vi "Menu_Property Node.vi"(11 "Affected Items Out":T1) -> (3 "Menu Items To Add":T2(array[cluster]))   [LabVIEW 2023]
uses:
  top/BundleMagic.ctl
  controls/action enum.ctl
panel:
  out "element":refnum<vi>
  out "Enabled Status":enum8{"Enabled", "Disabled"}[](array[ring])
  out "Menu Item Display Name":string[](array[string])
  out "Position In Menu":T3(array[cluster])
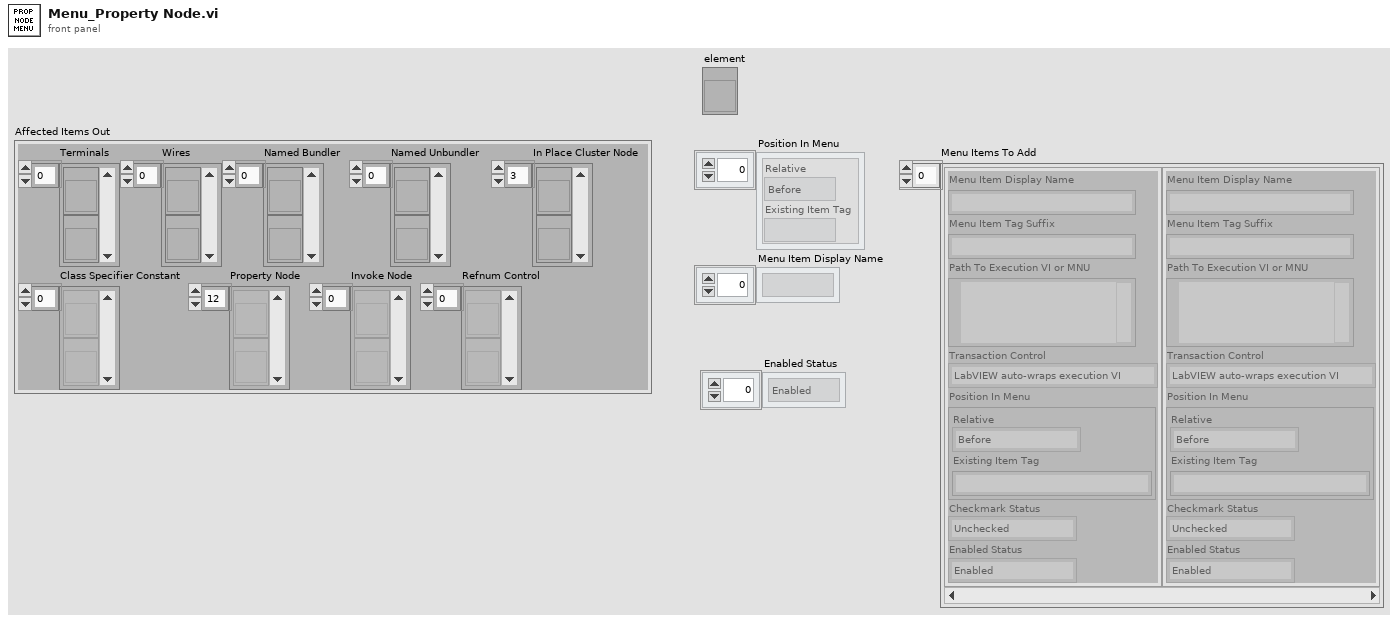
[diagram p1: front panel]
types:
  T1 = typedef "BundleMagic.ctl" = cluster{"Terminals":refnum<vi>[], "Wires":refnum<vi>[], "Named Bundler":refnum<vi>[], "Named Unbundler":refnum<vi>[], "In Place Cluster Node":refnum<vi>[], "Class Specifier Constant":refnum<vi>[], "Property Node":refnum<vi>[], "Invoke Node":refnum<vi>[], "Refnum Control":refnum<vi>[]}
  T2 = cluster{"Menu Item Display Name":string, "Menu Item Tag Suffix":string, "Path To Execution VI or MNU":path, "Transaction Control":enum8{"LabVIEW auto-wraps execution VI", "Execution VI will define if needed"}, "Position In Menu":cluster{"Relative":enum8{"Before", "Instead of", "After", "Into Submenu"}, "Existing Item Tag":string}, "Checkmark Status":enum8{"Unchecked", "Checked"}, "Enabled Status":enum8{"Enabled", "Disabled"}}[]
  T3 = cluster{"Relative":enum8{"Before", "Instead of", "After", "Into Submenu"}, "Existing Item Tag":string}[]
  T4 = typedef "action enum.ctl" = enum16{"[NONE]", "Wire Bundle", "Wire Unbundle", "Terminal Unbundle", "Terminal Bundle", "Bundler Move Up", "Bundler Move Down", "Bundler Insert", "Bundler Remove", "Bundler Remove Unwired", "Bundler Rearrange", "In Place Insert", "In Place Remove", "In Place Remove Unwired", "In Place Rearrange", "Wire Properties", "Wire Method", "Terminal Properties", "Terminal Method", "Property Move Up", "Property Move Down", "Properties Insert", "Properties Remove", "Properties Remove Unwired", "Properties Rearrange", "Method Change", "Class for Constant", "Class For Control", "Class For Node", "Class Name to Clipboard"}
  T5 = cluster{"Menu Item Display Name":string, "Menu Item Tag Suffix":string, "Path To Execution VI or MNU":path, "Transaction Control":enum8{"LabVIEW auto-wraps execution VI", "Execution VI will define if needed"}, "Position In Menu":cluster{"Relative":enum8{"Before", "Instead of", "After", "Into Submenu"}, "Existing Item Tag":string}, "Checkmark Status":enum8{"Unchecked", "Checked"}, "Enabled Status":enum8{"Enabled", "Disabled"}}
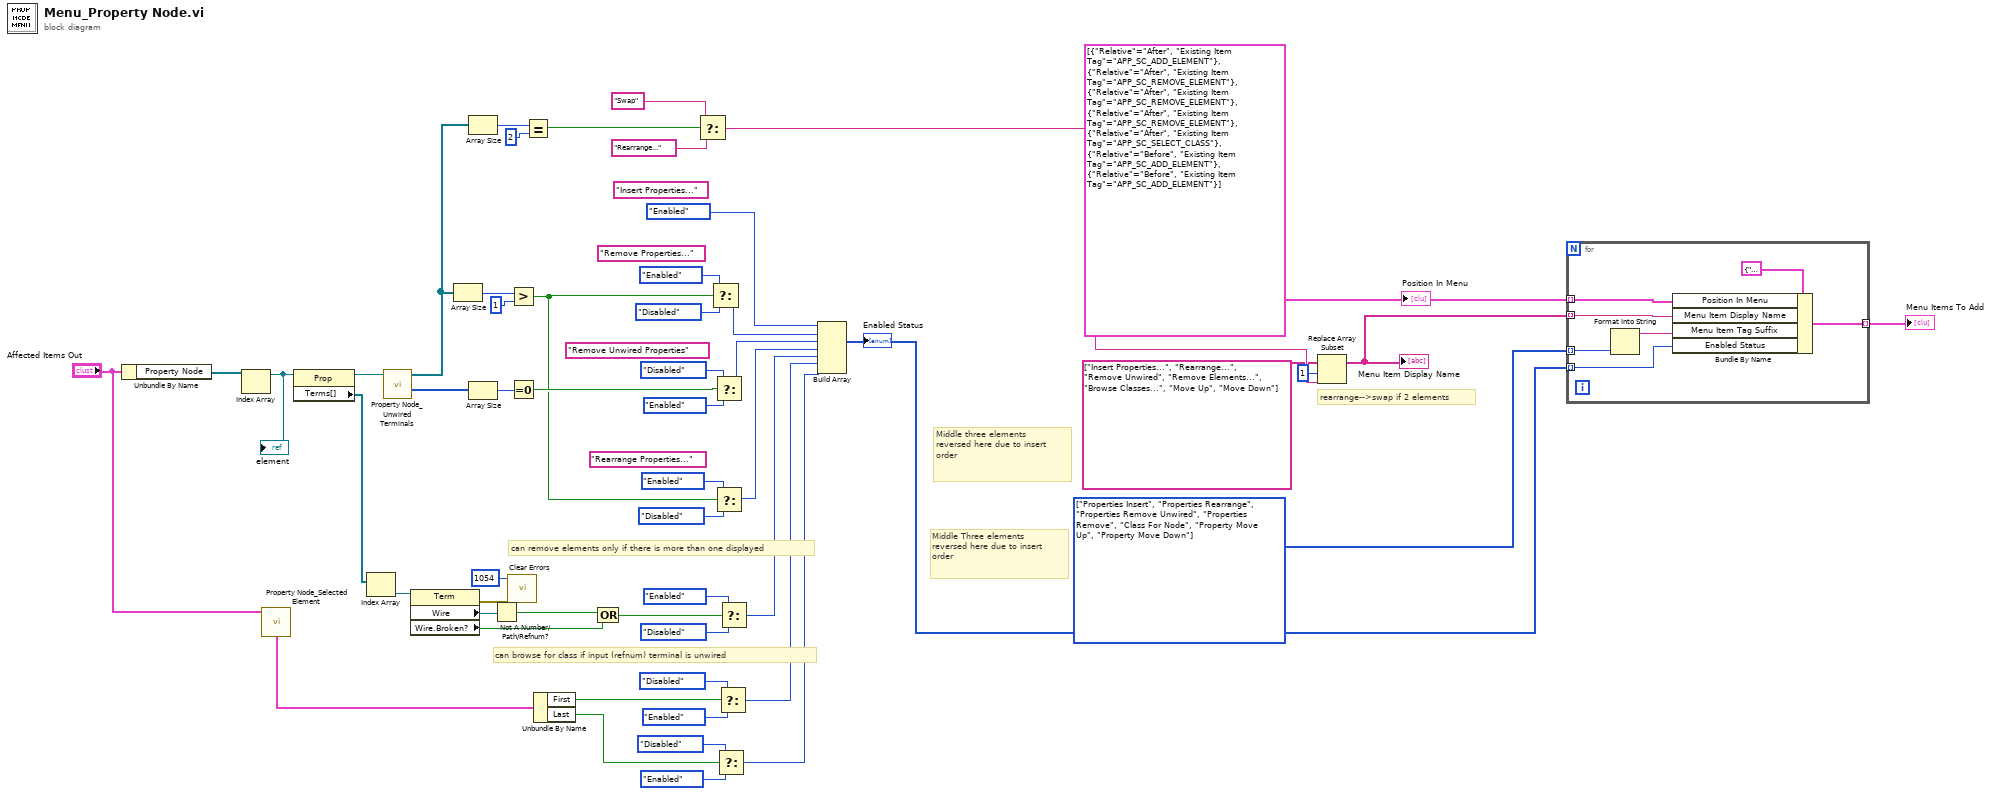
[diagram p0: block diagram]
diagram:
  (unwired) "Rearrange Properties..." ("Menu Item Display Name")
  (unwired) "Remove Unwired Properties" ("Menu Item Display Name")
  (unwired) "Remove Properties..." ("Menu Item Display Name")
  (unwired) "Insert Properties..." ("Menu Item Display Name")
  w54 = T3 [{"Relative"=enum."After", "Existing Item Tag"="APP_SC_ADD_ELEMENT"}, {"Relative"=enum."After", "Existing Item Tag"="APP_SC_REMOVE_ELEMENT"}, {"Relative"=enum."After", "Existing Item Tag"="APP_SC_REMOVE_ELEMENT"}, {"Relative"=enum."After", "Existing Item Tag"="APP_SC_REMOVE_ELEMENT"}, {"Relative"=enum."After", "Existing Item Tag"="APP_SC_SELECT_CLASS"}, {"Relative"=enum."Before", "Existing Item Tag"="APP_SC_ADD_ELEMENT"}, {"Relative"=enum."Before", "Existing Item Tag"="APP_SC_ADD_ELEMENT"}]
  w53 = T4[] [enum."Properties Insert", enum."Properties Rearrange", enum."Properties Remove Unwired", enum."Properties Remove", enum."Class For Node", enum."Property Move Up", enum."Property Move Down"] items=["[NONE]", "Wire Bundle", "Wire Unbundle", "Terminal Unbundle", "Terminal Bundle", "Bundler Move Up", "Bundler Move Down", "Bundler Insert", "Bundler Remove", "Bundler Remove Unwired", "Bundler Rearrange", "In Place Insert", "In Place Remove", "In Place Remove Unwired", "In Place Rearrange", "Wire Properties", "Wire Method", "Terminal Properties", "Terminal Method", "Property Move Up", "Property Move Down", "Properties Insert", "Properties Remove", "Properties Remove Unwired", "Properties Rearrange", "Method Change", "Class for Constant", "Class For Control", "Class For Node", "Class Name to Clipboard"]
  # "rearrange-->swap if 2 elements"
  # "can remove elements only if there is more than one displayed"
  # "can browse for class if input (refnum) terminal is unwired"
  # "Middle Three elements reversed here due to insert order"
  # "Middle three elements reversed here due to insert order"
  n1 = Unbundle By Name("Affected Items Out") -> ("Property Node"=w51:refnum<vi>[])
  n2 = Index Array(array=w51) -> (element=w21:refnum<vi>)  [unwired: 1 in]
  "element" <- w21
  n3 = call "Property Node_Selected Element.vi"("Affected Items"="Affected Items Out") -> ("Element details"=w19:cluster{"First":bool, "Last":bool})  [unwired: 5 in, 5 out]
  n4 = property class="Prop"(reference=w21) -> (reference out=w40:refnum<vi>, "Terms[]"=w48:refnum<vi>[])  [unwired: 1 in, 1 out]
  n5 = Index Array(array=w48) -> (element=w47:refnum<vi>)  [unwired: 1 in]
  n6 = call "Property Node_Unwired Terminals.vi"("Property Node Ref"=w40) -> ("Unwired Indices For Removal"=w32:i32[], "Property Items[]"=w7:refnum<vi>[])  [unwired: 7 in, 2 out]
  n7 = property class="Term"(reference=w47) -> (error out=w28:errorcluster, "Wire"=w46:refnum<vi>, "Wire.Broken?"=w31:bool)  [unwired: 1 in, 1 out]
  n8 = Array Size(array=w7) -> (size(s)=w50:i32)
  n9 = Array Size(array=w7) -> (size(s)=w9:i32)
  n10 = Array Size(array=w32) -> (size(s)=w38:i32)
  n11 = Not A Number/Path/Refnum?(number/path/refnum=w46) -> (NaN/Path/Refnum?=w30:bool)
  n12 = call <vilib>:"Clear Errors.vi"("error in (no error)"=w28, "specific error code to clear (0: all)"=1054) -> ()  [unwired: 4 in, 2 out]
  n13 = Greater?(x=w50, y=1) -> (0:w22:bool)
  n14 = Equal To 0?(x=w38) -> (x = 0?=w37:bool)
  n15 = Equal?(x=w9, y=2) -> (x = y?=w8:bool)
  n16 = Unbundle By Name(w19) -> ("First"=w14:bool, "Last"=w13:bool)
  n17 = Compound Arithmetic op=OR(w30, w31) -> (w29:bool)
  n18 = Select(t="Swap" ("Menu Item Display Name"), s=w8, f="Rearrange..." ("Menu Item Display Name")) -> (s? t:f=w3:string)
  n19 = Select(t=enum8{"Enabled", "Disabled"}."Enabled" ("Enabled Status"), s=w22, f=enum8{"Enabled", "Disabled"}."Disabled" ("Enabled Status")) -> (s? t:f=w23:enum8{"Enabled", "Disabled"})
  n20 = Select(t=enum8{"Enabled", "Disabled"}."Disabled" ("Enabled Status"), s=w37, f=enum8{"Enabled", "Disabled"}."Enabled" ("Enabled Status")) -> (s? t:f=w34:enum8{"Enabled", "Disabled"})
  n21 = Select(t=enum8{"Enabled", "Disabled"}."Enabled" ("Enabled Status"), s=w22, f=enum8{"Enabled", "Disabled"}."Disabled" ("Enabled Status")) -> (s? t:f=w39:enum8{"Enabled", "Disabled"})
  n22 = Select(t=enum8{"Enabled", "Disabled"}."Disabled" ("Enabled Status"), s=w13, f=enum8{"Enabled", "Disabled"}."Enabled" ("Enabled Status")) -> (s? t:f=w11:enum8{"Enabled", "Disabled"})
  n23 = Select(t=enum8{"Enabled", "Disabled"}."Disabled" ("Enabled Status"), s=w14, f=enum8{"Enabled", "Disabled"}."Enabled" ("Enabled Status")) -> (s? t:f=w12:enum8{"Enabled", "Disabled"})
  n24 = Select(t=enum8{"Enabled", "Disabled"}."Enabled" ("Enabled Status"), s=w29, f=enum8{"Enabled", "Disabled"}."Disabled" ("Enabled Status")) -> (s? t:f=w41:enum8{"Enabled", "Disabled"})
  n25 = Build Array(enum8{"Enabled", "Disabled"}."Enabled" ("Enabled Status"), w23, w34, w39, w41, w12, w11) -> (w33:enum8{"Enabled", "Disabled"}[])
  "Enabled Status" <- w33
  n26 = Replace Array Subset(array=string[] ["Insert Properties...", "Rearrange...", "Remove Unwired", "Remove Elements...", "Browse Classes...", "Move Up", "Move Down"], new element=w3, index=1) -> (w1:string[])
  "Menu Item Display Name" <- w1
  n27 = for {
    tunnel: [w61] -> w52 mode=indexing
    tunnel: w1 -> [w60] mode=indexing
    tunnel: w53 -> [w55] mode=indexing
    tunnel: w54 -> [w58] mode=indexing
    tunnel: w33 -> [w57] mode=indexing
    n28 = Format Into String(w55) -> (resulting string=w56:string)  [unwired: 3 in, 1 out]
    n29 = Bundle By Name(cluster=T5 {"Menu Item Display Name"="", "Menu Item Tag Suffix"="", "Path To Execution VI or MNU"=path "", "Transaction Control"=enum."LabVIEW auto-wraps execution VI", "Position In Menu"={"Relative"=enum."Before", "Existing Item Tag"=""}, "Checkmark Status"=enum."Unchecked", "Enabled Status"=enum."Enabled"} ("Cluster"), "Position In Menu"=w58, "Menu Item Display Name"=w60, "Menu Item Tag Suffix"=w56, "Enabled Status"=w57) -> (w61:T5)
  }
  "Menu Items To Add" <- w52
  "Position In Menu" <- w54
